vi "MainPubSub.vi"() -> ()   [LabVIEW 2018]
uses:
  <vilib>/addons/zeromq/zmq_context.lvclass
  socket REQ/socket REQ.lvclass
  socket REP/socket REP.lvclass
  socket SUB/socket SUB.lvclass
  C:/Users/Denis/Desktop/communication-manager/communication-manager/Socket/Socket.lvclass
  RxTx/RxTx.lvclass
  Socket/Socket.lvclass
panel:
  in  "socket SUB.lvclass":refnum<class "socket SUB.lvclass">
  in  "socket REP.lvclass":refnum<class "socket REP.lvclass">
  in  "socket REQ.lvclass":refnum<class "socket REQ.lvclass">
  out "context":refnum<class "zmq_context.lvclass">
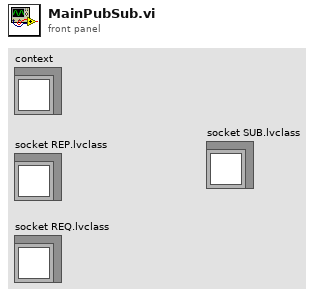
[diagram p1: front panel]
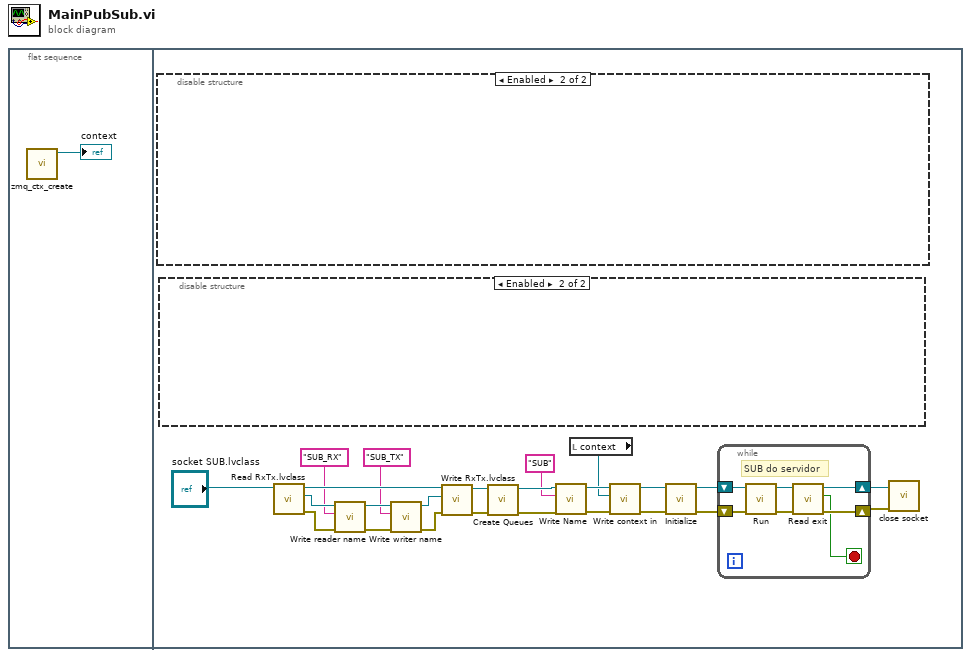
[diagram p0: block diagram]
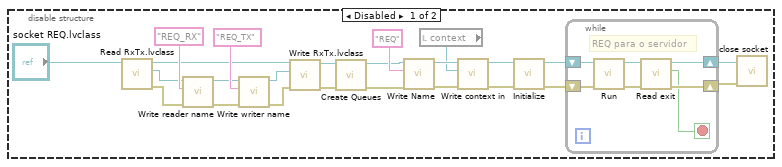
[diagram p2: hidden frame]
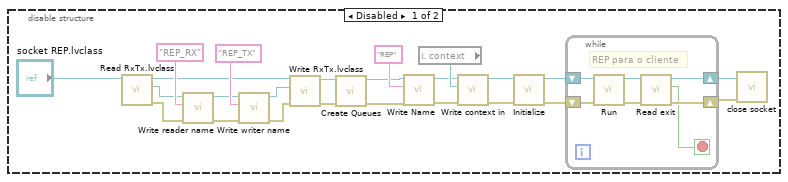
[diagram p3: hidden frame]
diagram:
  n1 = flat-sequence {
    frame #0 {
      n2 = call <vilib>:"zmq_ctx_create.vi"() -> ("context out"=→"context":refnum<class "zmq_context.lvclass">)  [unwired: 4 in, 1 out]
    }
    frame #1 {
      n3 = disable-structure shown="Enabled" {
        frame Disabled {
          n4 = call-dynamic "Read RxTx.lvclass.vi"("Socket in"="socket REP.lvclass") -> ("error out"=w72:errorcluster, "RxTx.lvclass"=w78:refnum<class "RxTx.lvclass">, "Socket out"=w75:refnum<class "socket REP.lvclass">)  [unwired: 8 in]
          n5 = call-dynamic "Write reader name.vi"("error in (no error)"=w72, "RX name"="REP_RX" ("reader name"), "RxTx in"=w78) -> ("error out"=w71:errorcluster, "RxTx out"=w77:refnum<class "RxTx.lvclass">)  [unwired: 7 in]
          n6 = call-dynamic "Write writer name.vi"("error in (no error)"=w71, "Tx name"="REP_TX" ("writer name"), "RxTx in"=w77) -> ("error out"=w70:errorcluster, "RxTx out"=w76:refnum<class "RxTx.lvclass">)  [unwired: 7 in]
          n7 = call-dynamic "Write RxTx.lvclass.vi"("error in (no error)"=w70, "RxTx.lvclass"=w76, "Socket in"=w75) -> ("error out"=w73:errorcluster, "Socket out"=w74:refnum<class "socket REP.lvclass">)  [unwired: 7 in]
          n8 = call-dynamic "Create Queues.vi"("error in (no error)"=w73, "Socket in"=w74) -> ("error out"=w63:errorcluster, "Socket out"=w66:refnum<class "socket REP.lvclass">)  [unwired: 8 in]
          n9 = call-dynamic "Write Name.vi"("error in (no error)"=w63, "Name"="REP", "Socket in"=w66) -> ("error out"=w62:errorcluster, "Socket out"=w65:refnum<class "socket REP.lvclass">)  [unwired: 7 in]
          n10 = local read "context"() -> (w67:refnum<class "zmq_context.lvclass">)
          n11 = call-dynamic "Write context in.vi"("error in (no error)"=w62, "zeromq.lvlib:ZeroMQ Context"=w67, "Socket in"=w65) -> ("error out"=w61:errorcluster, "Socket out"=w64:refnum<class "socket REP.lvclass">)  [unwired: 7 in]
          n12 = call-dynamic "Initialize.vi"("error in (no error)"=w61, "socket REP in"=w64) -> ("error out"=w58:errorcluster, "socket REP out"=w60:refnum<class "socket REP.lvclass">)  [unwired: 8 in]
          n13 = while {
            shift-right: [w85] -> w59
            shift-left: w60 -> [w87]
            shift-right: [w82] -> w57
            shift-left: w58 -> [w84]
            stop <- w81 stop-if-true
            # "REP para o cliente"
            n14 = call-dynamic "Run.vi"("error in (no error)"=w84, "socket REP in"=w87) -> ("error out"=w83:errorcluster, "socket REP out"=w86:refnum<class "socket REP.lvclass">)  [unwired: 8 in]
            n15 = call-dynamic "Read exit.vi"("error in (no error)"=w83, "Socket in"=w86) -> ("error out"=w82:errorcluster, "exit"=w81:bool, "Socket out"=w85:refnum<class "socket REP.lvclass">)  [unwired: 7 in]
          }
          n16 = call "close socket.vi"("error in (no error)"=w57, "Socket in"=w59) -> ()  [unwired: 8 in, 2 out]
        }
        frame Enabled {
        }
      }
      n17 = disable-structure shown="Enabled" {
        frame Disabled {
          n18 = call-dynamic "Read RxTx.lvclass.vi"("Socket in"="socket REQ.lvclass") -> ("error out"=w41:errorcluster, "RxTx.lvclass"=w47:refnum<class "RxTx.lvclass">, "Socket out"=w44:refnum<class "socket REQ.lvclass">)  [unwired: 8 in]
          n19 = call-dynamic "Write reader name.vi"("error in (no error)"=w41, "RX name"="REQ_RX" ("reader name"), "RxTx in"=w47) -> ("error out"=w40:errorcluster, "RxTx out"=w46:refnum<class "RxTx.lvclass">)  [unwired: 7 in]
          n20 = call-dynamic "Write writer name.vi"("error in (no error)"=w40, "Tx name"="REQ_TX" ("writer name"), "RxTx in"=w46) -> ("error out"=w39:errorcluster, "RxTx out"=w45:refnum<class "RxTx.lvclass">)  [unwired: 7 in]
          n21 = call-dynamic "Write RxTx.lvclass.vi"("error in (no error)"=w39, "RxTx.lvclass"=w45, "Socket in"=w44) -> ("error out"=w42:errorcluster, "Socket out"=w43:refnum<class "socket REQ.lvclass">)  [unwired: 7 in]
          n22 = call-dynamic "Create Queues.vi"("error in (no error)"=w42, "Socket in"=w43) -> ("error out"=w34:errorcluster, "Socket out"=w37:refnum<class "socket REQ.lvclass">)  [unwired: 8 in]
          n23 = call-dynamic "Write Name.vi"("error in (no error)"=w34, "Name"="REQ", "Socket in"=w37) -> ("error out"=w33:errorcluster, "Socket out"=w36:refnum<class "socket REQ.lvclass">)  [unwired: 7 in]
          n24 = local read "context"() -> (w26:refnum<class "zmq_context.lvclass">)
          n25 = call-dynamic "Write context in.vi"("error in (no error)"=w33, "zeromq.lvlib:ZeroMQ Context"=w26, "Socket in"=w36) -> ("error out"=w32:errorcluster, "Socket out"=w35:refnum<class "socket REQ.lvclass">)  [unwired: 7 in]
          n26 = call-dynamic "Initialize.vi"("error in (no error)"=w32, "socket REQ in"=w35) -> ("error out"=w29:errorcluster, "socket REQ out"=w31:refnum<class "socket REQ.lvclass">)  [unwired: 8 in]
          n27 = while {
            shift-right: [w54] -> w30
            shift-left: w31 -> [w56]
            shift-right: [w51] -> w28
            shift-left: w29 -> [w53]
            stop <- w50 stop-if-true
            # "REQ para o servidor"
            n28 = call-dynamic "Run.vi"("error in (no error)"=w53, "socket REQ in"=w56) -> ("error out"=w52:errorcluster, "socket REQ out"=w55:refnum<class "socket REQ.lvclass">)  [unwired: 8 in]
            n29 = call-dynamic "Read exit.vi"("error in (no error)"=w52, "Socket in"=w55) -> ("error out"=w51:errorcluster, "exit"=w50:bool, "Socket out"=w54:refnum<class "socket REQ.lvclass">)  [unwired: 7 in]
          }
          n30 = call "close socket.vi"("error in (no error)"=w28, "Socket in"=w30) -> ()  [unwired: 8 in, 2 out]
        }
        frame Enabled {
        }
      }
      n31 = call-dynamic "Read RxTx.lvclass.vi"("Socket in"="socket SUB.lvclass") -> ("error out"=w12:errorcluster, "RxTx.lvclass"=w6:refnum<class "RxTx.lvclass">, "Socket out"=w9:refnum<class "socket SUB.lvclass">)  [unwired: 8 in]
      n32 = call-dynamic "Write reader name.vi"("error in (no error)"=w12, "RX name"="SUB_RX" ("reader name"), "RxTx in"=w6) -> ("error out"=w13:errorcluster, "RxTx out"=w7:refnum<class "RxTx.lvclass">)  [unwired: 7 in]
      n33 = call-dynamic "Write writer name.vi"("error in (no error)"=w13, "Tx name"="SUB_TX" ("writer name"), "RxTx in"=w7) -> ("error out"=w14:errorcluster, "RxTx out"=w8:refnum<class "RxTx.lvclass">)  [unwired: 7 in]
      n34 = call-dynamic "Write RxTx.lvclass.vi"("error in (no error)"=w14, "RxTx.lvclass"=w8, "Socket in"=w9) -> ("error out"=w11:errorcluster, "Socket out"=w10:refnum<class "socket SUB.lvclass">)  [unwired: 7 in]
      n35 = call-dynamic "Create Queues.vi"("error in (no error)"=w11, "Socket in"=w10) -> ("error out"=w19:errorcluster, "Socket out"=w16:refnum<class "socket SUB.lvclass">)  [unwired: 8 in]
      n36 = call-dynamic "Write Name.vi"("error in (no error)"=w19, "Name"="SUB", "Socket in"=w16) -> ("error out"=w20:errorcluster, "Socket out"=w17:refnum<class "socket SUB.lvclass">)  [unwired: 7 in]
      n37 = local read "context"() -> (w3:refnum<class "zmq_context.lvclass">)
      n38 = call-dynamic "Write context in.vi"("error in (no error)"=w20, "zeromq.lvlib:ZeroMQ Context"=w3, "Socket in"=w17) -> ("error out"=w21:errorcluster, "Socket out"=w18:refnum<class "socket SUB.lvclass">)  [unwired: 7 in]
      n39 = call-dynamic "Initialize.vi"("error in (no error)"=w21, "socket SUB in"=w18) -> ("error out"=w24:errorcluster, "socket SUB out"=w22:refnum<class "socket SUB.lvclass">)  [unwired: 8 in]
      n40 = while {
        shift-right: [w92] -> w23
        shift-left: w22 -> [w94]
        shift-right: [w89] -> w25
        shift-left: w24 -> [w91]
        stop <- w88 stop-if-true
        # "SUB do servidor"
        n41 = call-dynamic "Run.vi"("error in (no error)"=w91, "socket SUB in"=w94) -> ("error out"=w90:errorcluster, "socket SUB out"=w93:refnum<class "socket SUB.lvclass">)  [unwired: 8 in]
        n42 = call-dynamic "Read exit.vi"("error in (no error)"=w90, "Socket in"=w93) -> ("error out"=w89:errorcluster, "exit"=w88:bool, "Socket out"=w92:refnum<class "socket SUB.lvclass">)  [unwired: 7 in]
      }
      n43 = call "close socket.vi"("error in (no error)"=w25, "Socket in"=w23) -> ()  [unwired: 8 in, 2 out]
    }
  }
